vi "U64ToI64.vi"(5 "Number":u64) -> (1 "Signed 64-bit integer":i64, 2 "Overflow?":bool, 3 "Exact conversion?":bool)   [LabVIEW 2017, in "GPOverflow.lvlib"]
doc: "Converts <B>Number</B> to I64 keeping track of numeric overflow and exactness of conversion.\n\n<B>Exact conversion?</B> will be True only if a conversion back into the original data type of <B>Number</B> will yield the exact same number, i.e. no precision was lost during the conversion.\n\n<B>Overflow?</B> will be True if positive or negative overflow occurred. The numeric output will saturate in case of overflow.\n\nThis VI is inlined.\n\nSteen Schmidt\nGPower\n6/3 2013"
uses:
  GPOverflow.lvlib
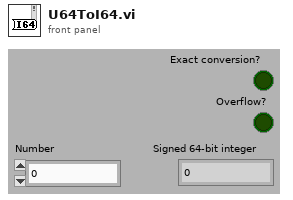
[diagram p1: front panel]
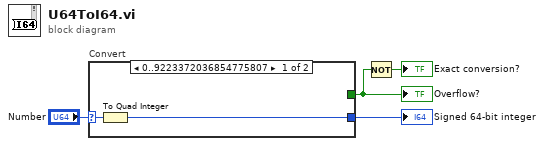
[diagram p0: block diagram]
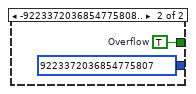
[diagram p2: hidden frame]
diagram:
  n1 = case "Convert" shown="0..9223372036854775807" "Number" {
    selector: "Number" -> [w6 _]
    tunnel: [w5 i64 9223372036854775807] -> w3
    tunnel: [_ w7] -> w2
    frame 0..9223372036854775807 {
      n2 = To Quad Integer(1:w6) -> (0:w5:i64)
    }
    frame -9223372036854775808.. {
      w7 = TRUE  # Overflow
    }
  }
  "Signed 64-bit integer" <- w3
  "Overflow?" <- w2
  n3 = Not(x=w2) -> (.not. x?=→"Exact conversion?":bool)
